vi "_dialog.vi"   [LabVIEW 2019]
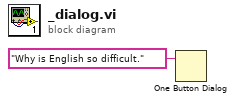
[diagram p0: block diagram]
diagram:
  n1 = One Button Dialog(message="Why is English so difficult." ("消息")) -> ()  [unwired: 1 in, 1 out]
